vi "AccessData.vi"(0 "Vibration_Channel4_FFT":refnum<queue>, 1 "Vibration_Channel3_FFT":refnum<queue>, 2 "Vibration_Channel2_FFT":refnum<queue>, 3 "Vibration_Channel1_FFT":refnum<queue>, 4 "Vibration_Channel1":refnum<queue>, 5 "Vibration_Channel2":refnum<queue>, 6 "Vibration_Channel3":refnum<queue>, 7 "Vibration_Channel4":refnum<queue>, 8 "created path":path, 9 "Speed_Channel":refnum<queue>, 10 "IP地址":string, 12 "PRE_Scaler":u8, 14 "SAVE?":bool, 16 "Sensitivity":u16=6554, 18 "Run":refnum<queue>, 20 "Temperature_Channel1":refnum<queue>, 21 "Temperature_Channel2":refnum<queue>, 22 "Temperature_Channel3":refnum<queue>, 23 "Temperature_Channel4":refnum<queue>, 24 "Temperature_Channel5":refnum<queue>, 25 "Temperature_Channel6":refnum<queue>, 26 "Temperature_Channel7":refnum<queue>, 27 "Humidity_Channel":refnum<queue>) -> ()   [LabVIEW 2012]
uses:
  <vilib>/Analysis/NI_AALPro.lvlib
panel:
  out "系统时间":string
  out "收包":i32
  out "KB/s":dbl
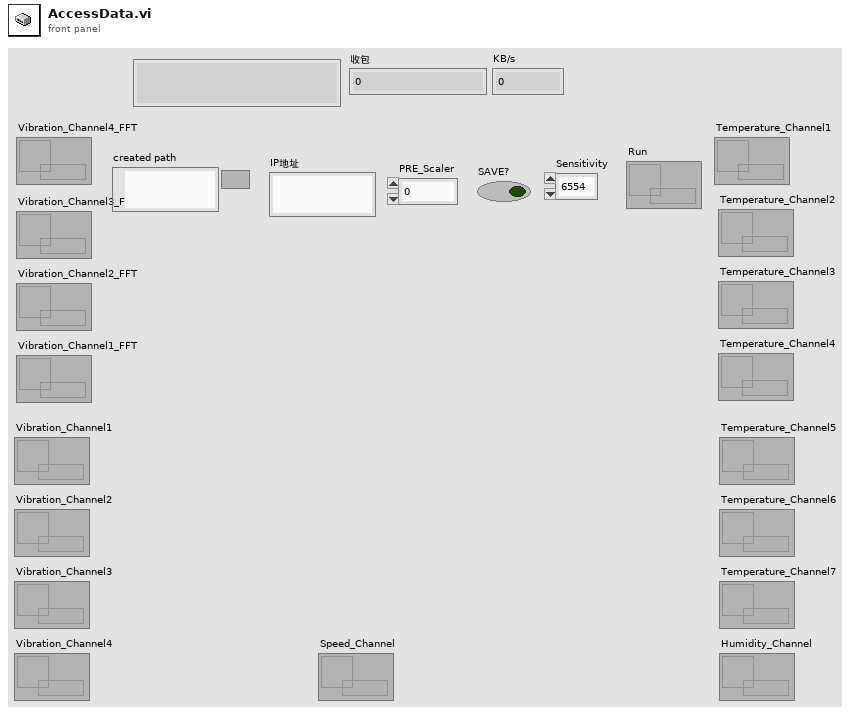
[diagram p1: front panel]
types:
  T1 = enum16{"open", "replace", "create", "open or create", "replace or create", "replace or create with confirmation"}
  T2 = enum16{"big-endian, network order", "native, host order", "little-endian"}
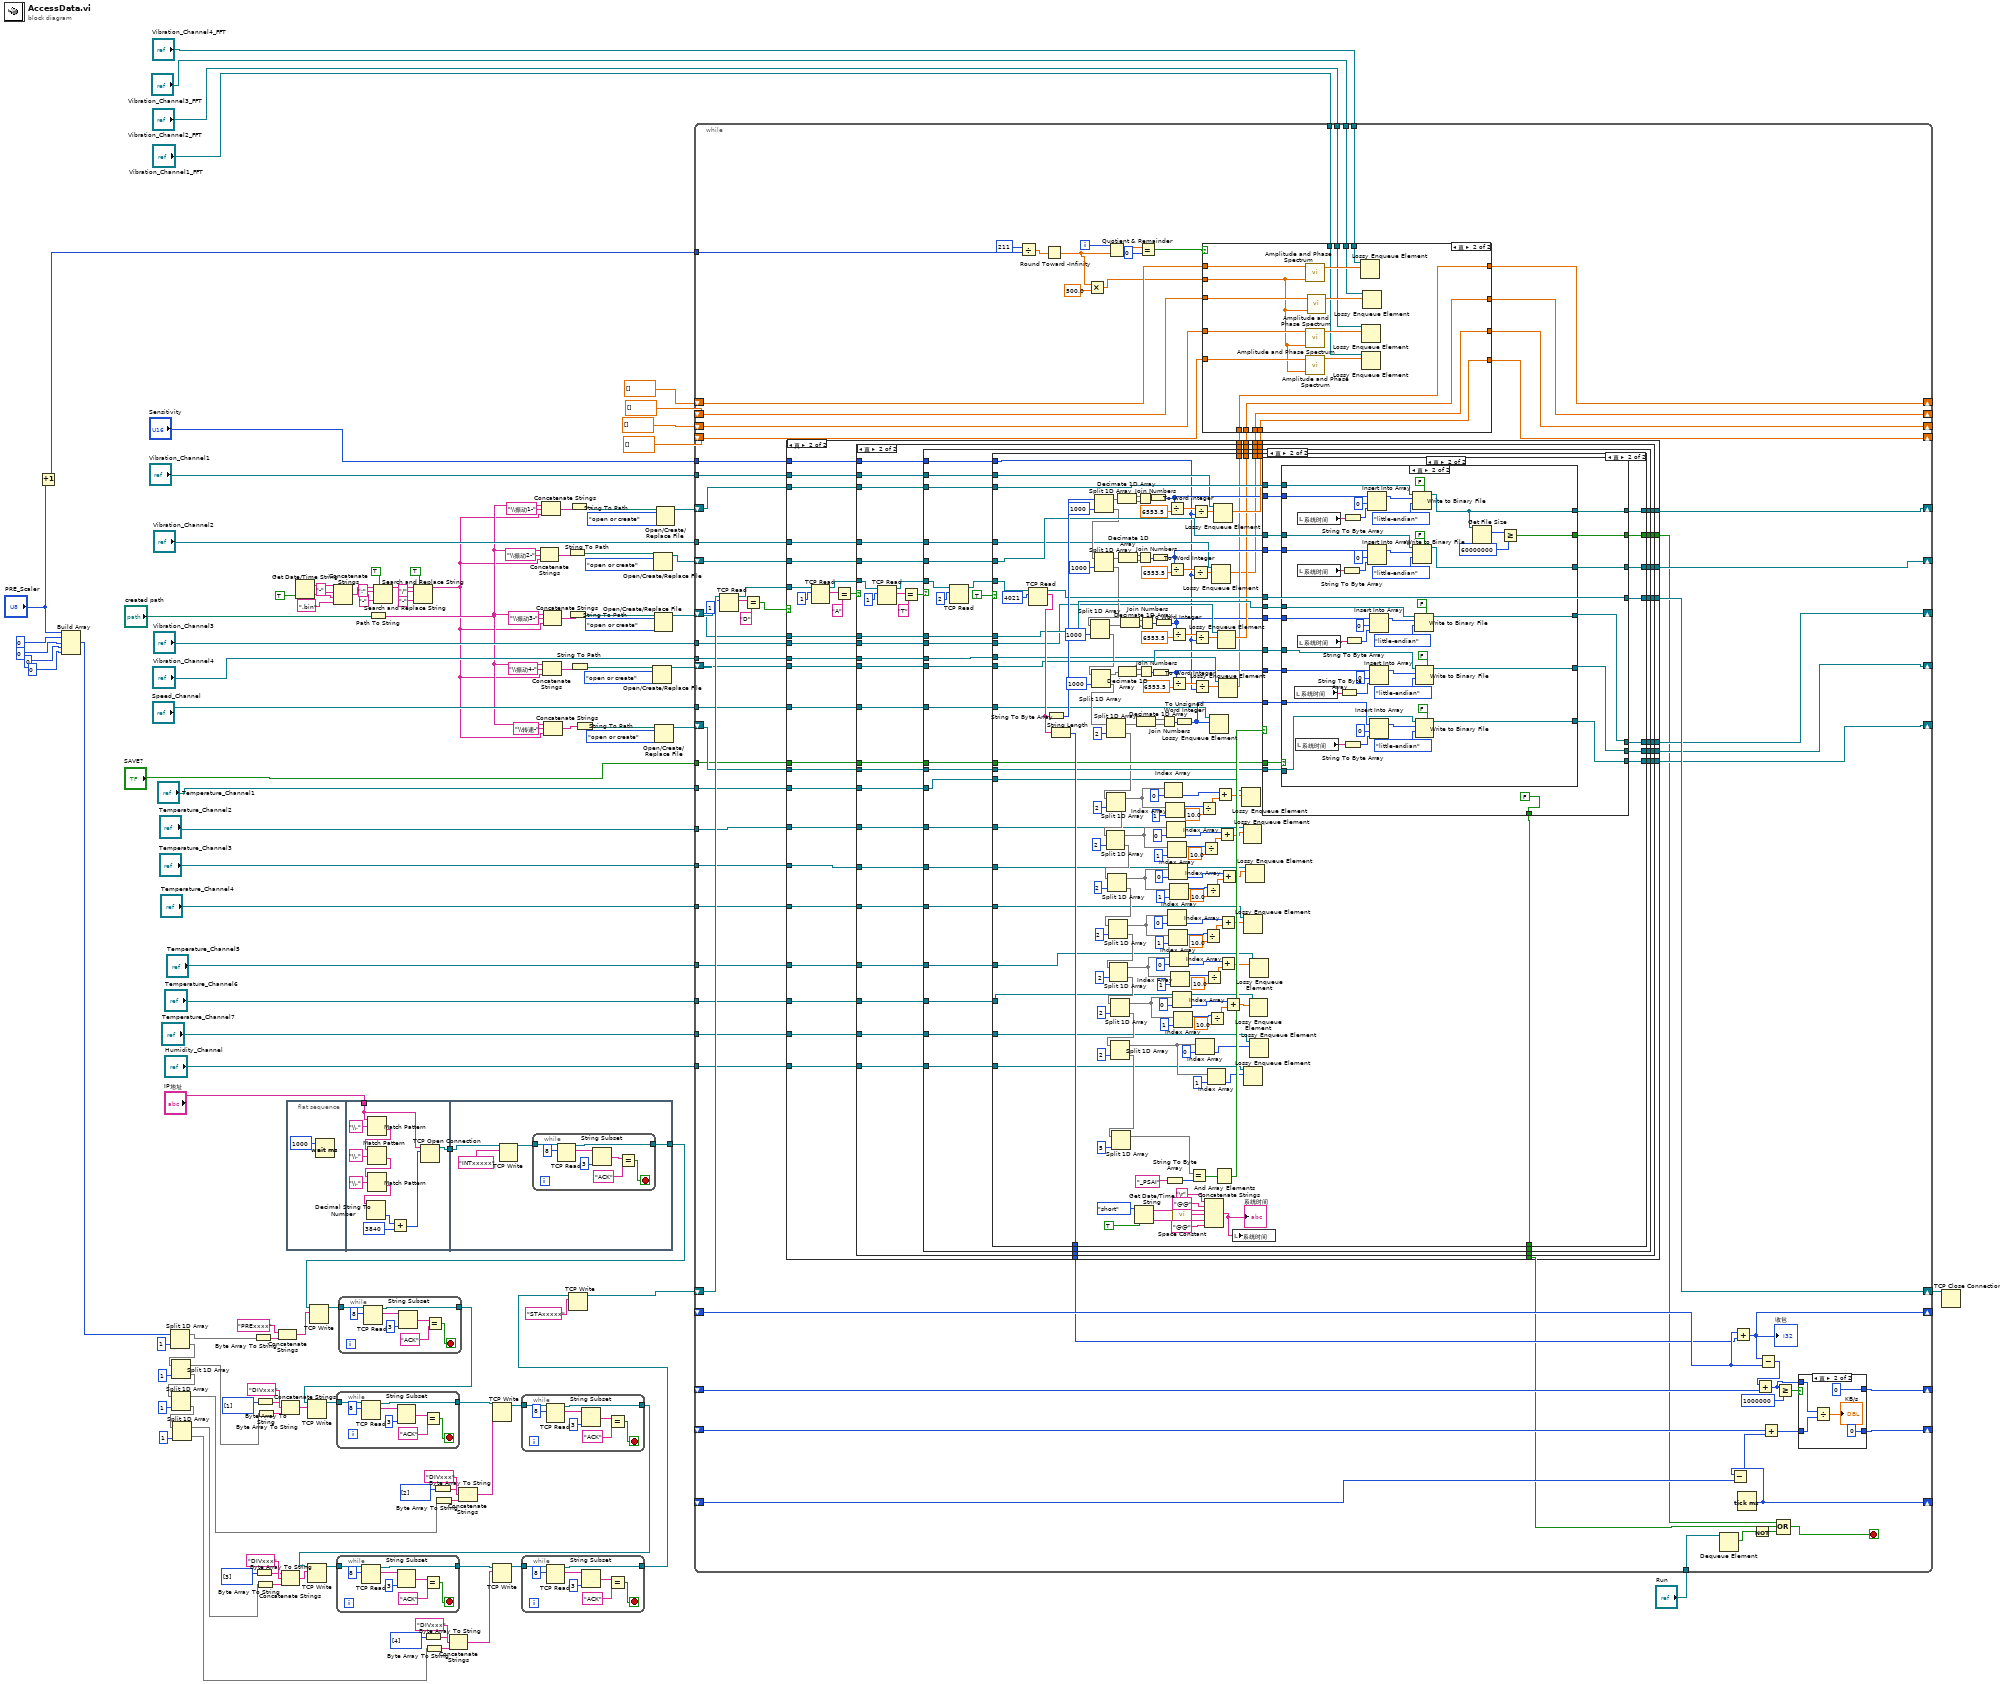
[diagram p0: block diagram]
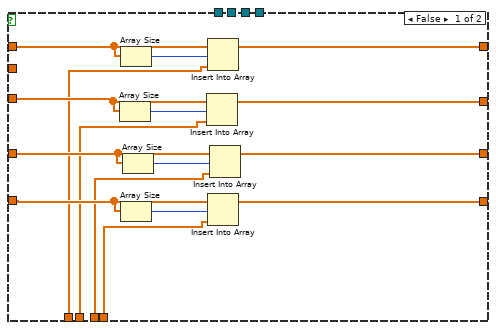
[diagram p2: hidden frame]
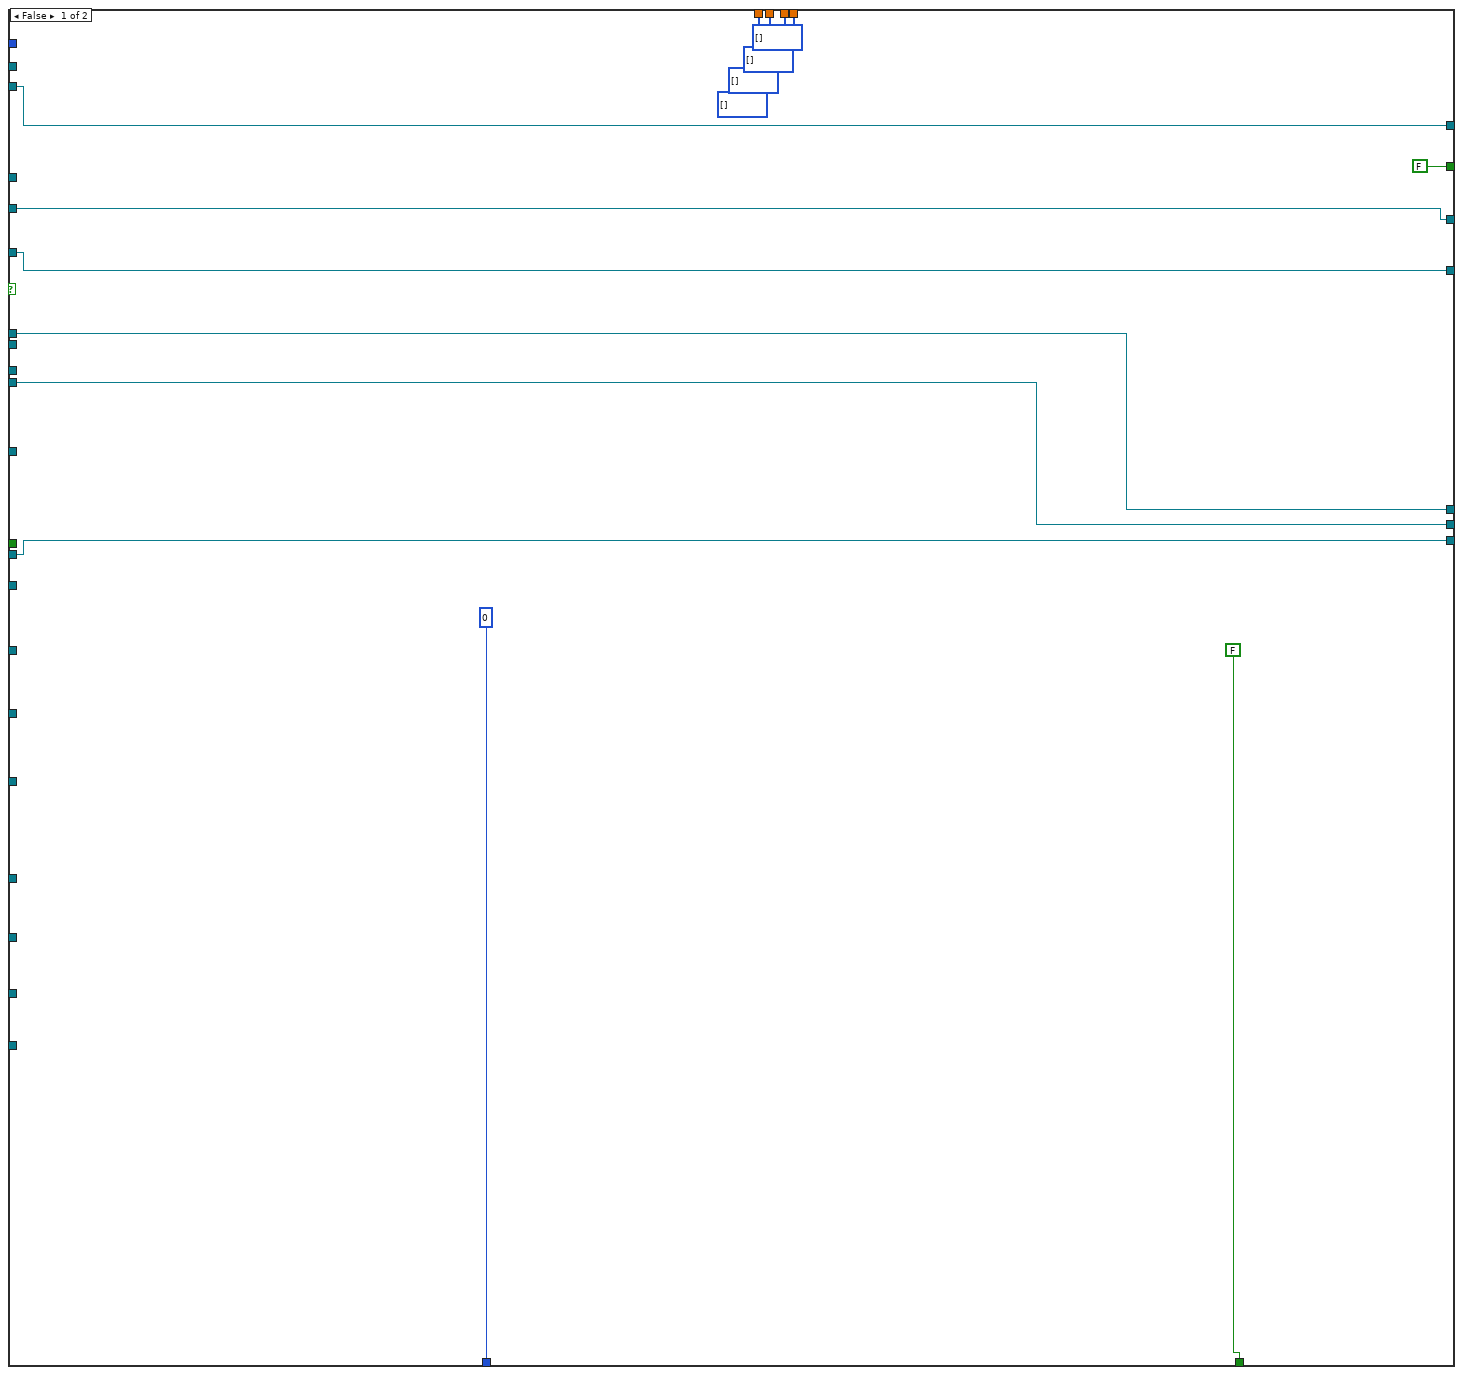
[diagram p3: hidden frame]
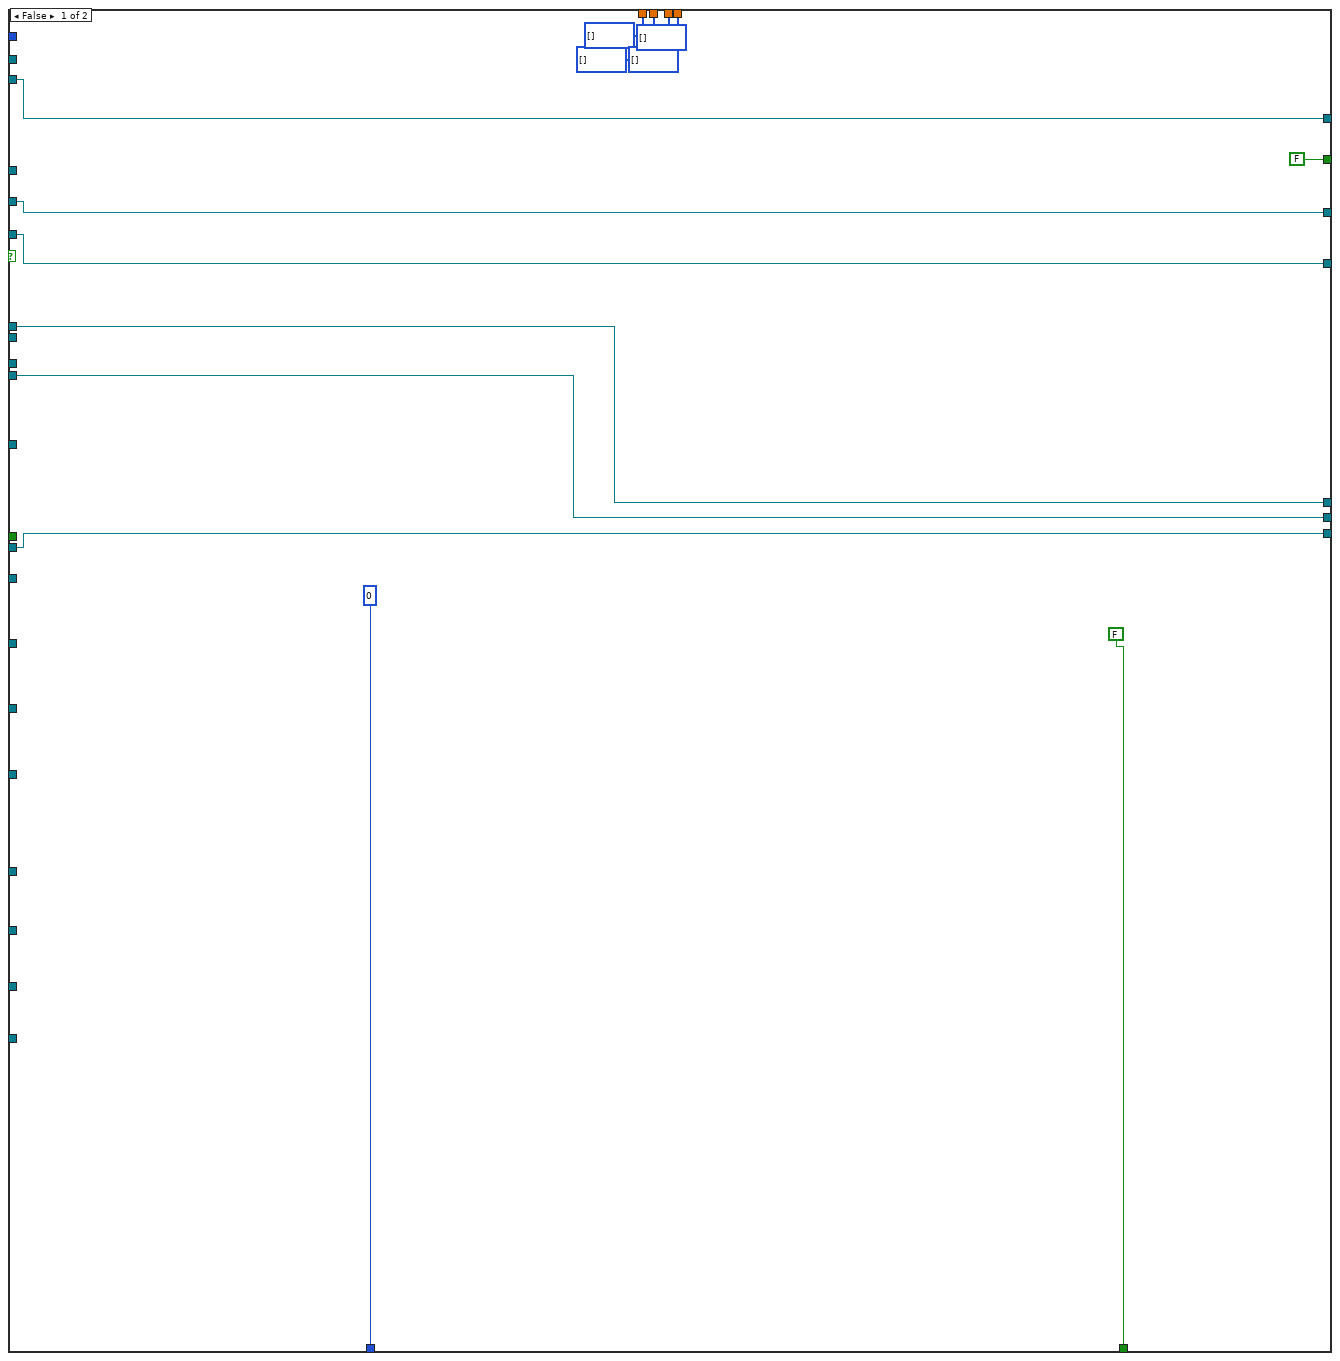
[diagram p4: hidden frame]
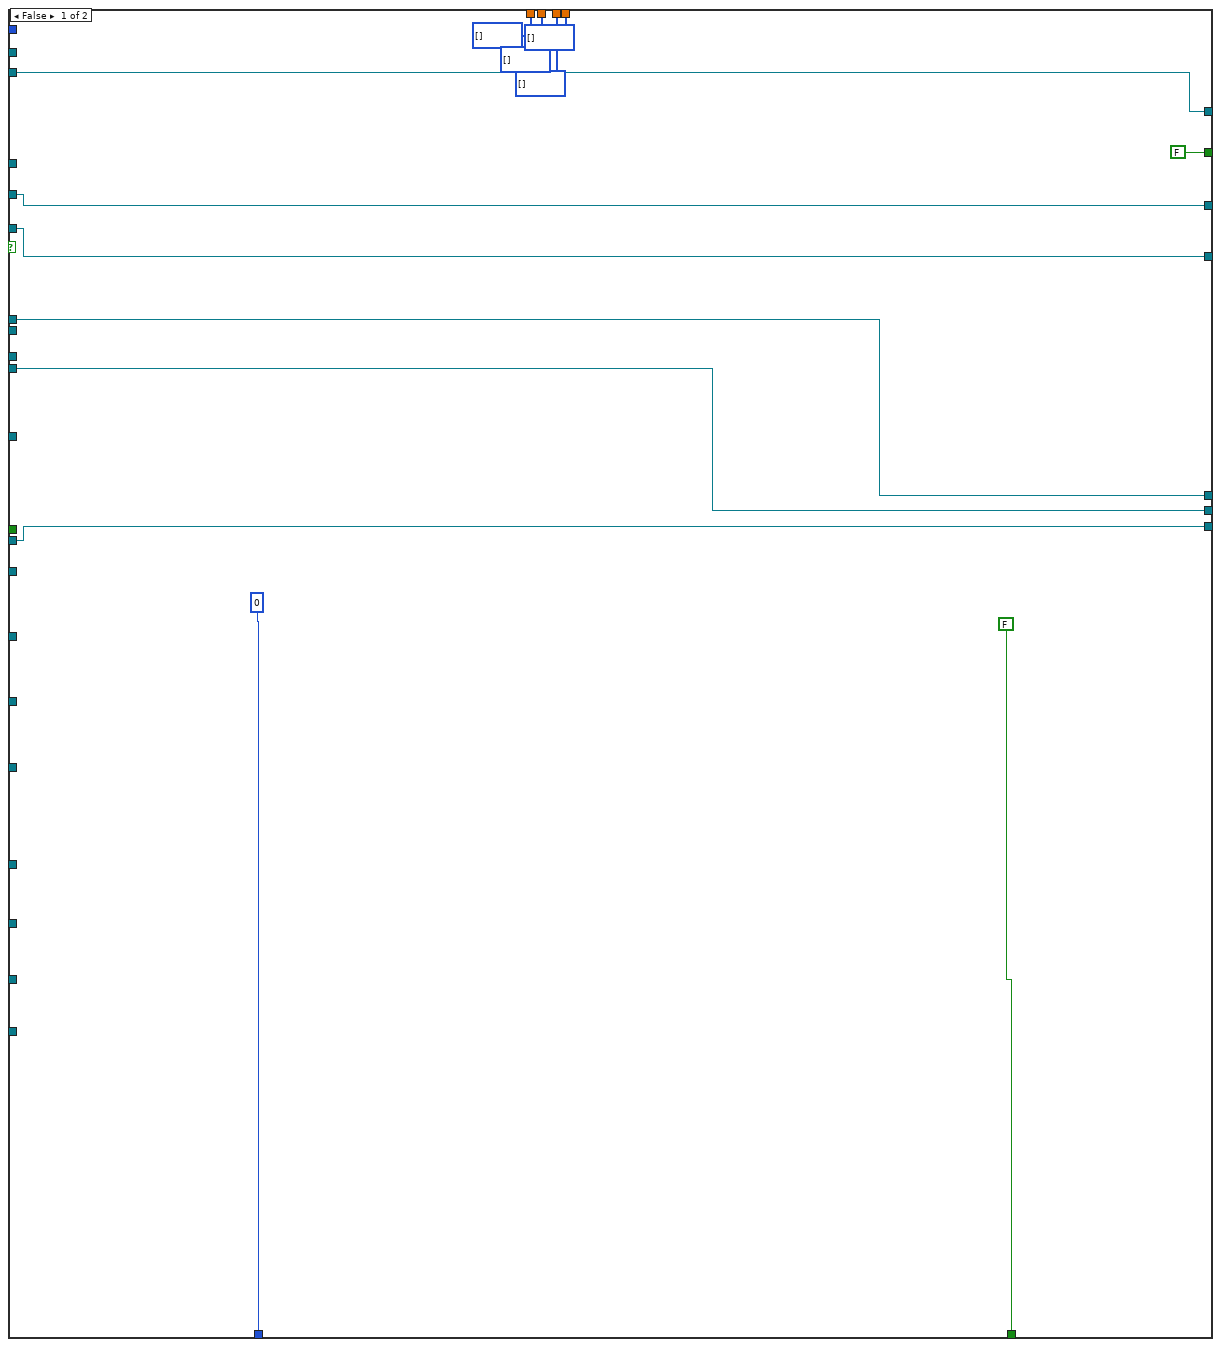
[diagram p5: hidden frame]
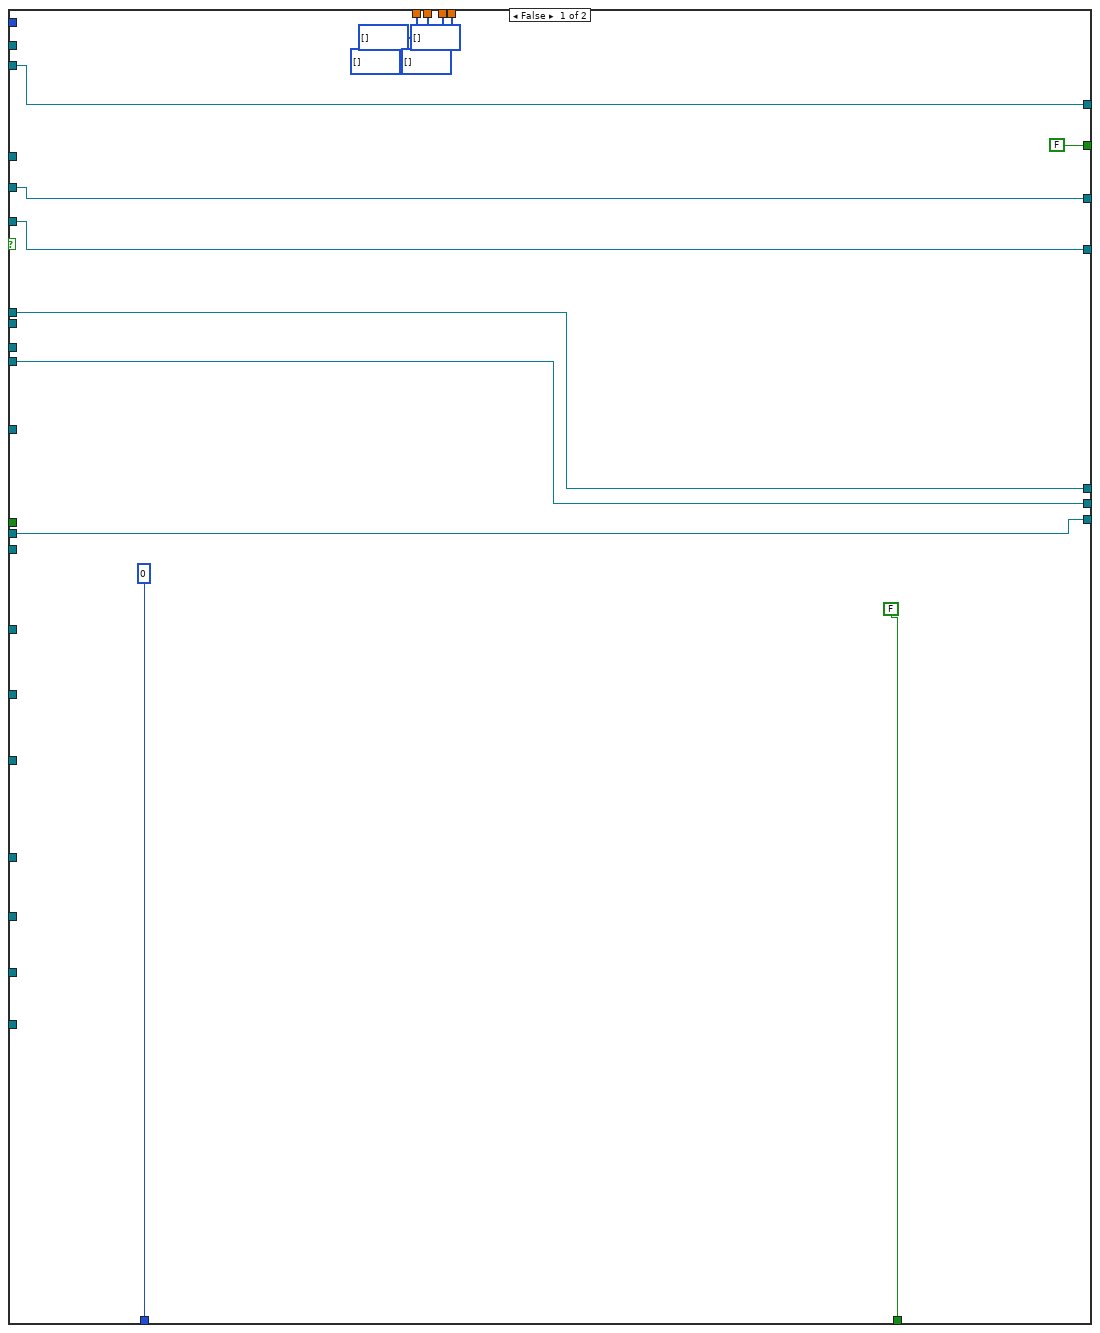
[diagram p6: hidden frame]
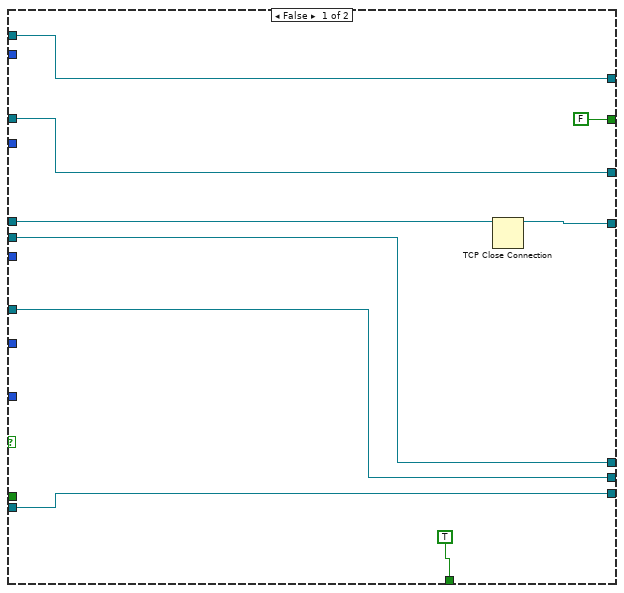
[diagram p7: hidden frame]
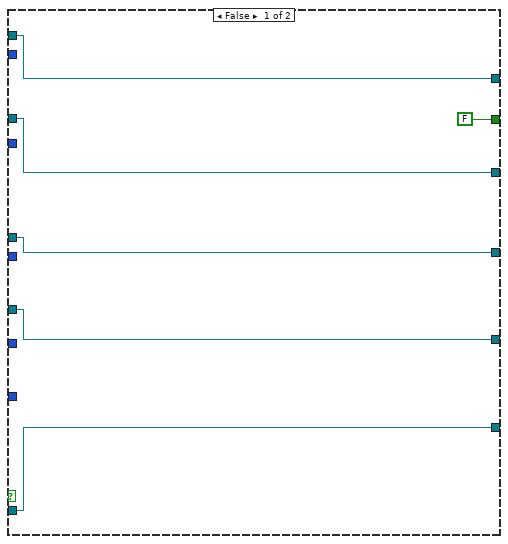
[diagram p8: hidden frame]
diagram:
  n1 = Increment(x="PRE_Scaler") -> (x+1=w101:u8)
  n2 = Build Array("PRE_Scaler", u8 0 ("元素"), u8 0 ("元素"), u8 0 ("元素"), u8 0 ("元素")) -> (w122:u8[])
  n3 = Split 1D Array(array=w122, index=1 ("索引")) -> (first subarray=w81:u8[], second subarray=w77:u8[])
  n4 = Split 1D Array(array=w77, index=1 ("索引")) -> (first subarray=w57:u8[], second subarray=w76:u8[])
  n5 = Split 1D Array(array=w76, index=1 ("索引")) -> (first subarray=w56:u8[], second subarray=w75:u8[])
  n6 = Split 1D Array(array=w75, index=1 ("索引")) -> (first subarray=w55:u8[], second subarray=w54:u8[])
  n7 = Byte Array To String(unsigned byte array=w81) -> (string=w85:string)
  n8 = Byte Array To String(unsigned byte array=u8[] [3] ("无符号字节数组")) -> (string=w63:string)
  n9 = Byte Array To String(unsigned byte array=u8[] [1] ("无符号字节数组")) -> (string=w71:string)
  n10 = Byte Array To String(unsigned byte array=w55) -> (string=w65:string)
  n11 = Byte Array To String(unsigned byte array=w57) -> (string=w74:string)
  n12 = Concatenate Strings("PRExxxx" ("数据输入"), w85) -> (w83:string)
  n13 = Concatenate Strings("DIVxxx" ("数据输入"), w71, w74) -> (w73:string)
  n14 = Concatenate Strings("DIVxxx" ("数据输入"), w63, w65) -> (w48:string)
  n15 = flat-sequence {
    tunnel: [w135] -> w123
    tunnel: "IP地址" -> [w126]
    tunnel: w123 -> [w138]
    tunnel: [w136] -> w47
    frame #0 {
      n16 = Wait (ms)(milliseconds to wait=u32 1000 ("毫秒倍数")) -> ()  [unwired: 1 out]
    }
    frame #1 {
      n17 = Match Pattern(string=w126, regular expression="\\." ("正则表达式")) -> (after substring=w130:string)  [unwired: 1 in, 3 out]
      n18 = Match Pattern(string=w130, regular expression="\\." ("正则表达式")) -> (after substring=w131:string)  [unwired: 1 in, 3 out]
      n19 = Match Pattern(string=w131, regular expression="\\." ("正则表达式")) -> (after substring=w132:string)  [unwired: 1 in, 3 out]
      n20 = Decimal String To Number(string=w132) -> (number=w133:i32)  [unwired: 2 in, 1 out]
      n21 = Add(x=w133, y=3840) -> (x+y=w125:i32)
      n22 = TCP Open Connection(address=w126, remote port or service name=w125) -> (connection ID=w135:refnum<k5>)  [unwired: 3 in, 1 out]
    }
    frame #2 {
      n23 = TCP Write(connection ID=w138, data in="INTxxxxx" ("数据输入")) -> (connection ID out=w137:refnum<k5>)  [unwired: 2 in, 2 out]
      n24 = while {
        tunnel: w137 -> [w147]
        tunnel: [w141] -> w136
        stop <- w142 stop-if-true
        n25 = TCP Read(connection ID=w147, bytes to read=8 ("读取的字节")) -> (connection ID out=w141:refnum<k5>, data out=w145:string)  [unwired: 3 in, 1 out]
        n26 = String Subset(string=w145, length (rest)=3 ("偏移量(0)")) -> (substring=w144:string)  [unwired: 1 in]
        n27 = Equal?(x=w144, y="ACK") -> (x = y?=w142:bool)
      }
    }
  }
  n28 = Get Date/Time String(want seconds? (F)=TRUE ("需要秒？(F)")) -> (date string=w19:string, time string=w16:string)  [unwired: 2 in]
  n29 = TCP Write(connection ID=w47, data in=w83) -> (connection ID out=w94:refnum<k5>)  [unwired: 2 in, 2 out]
  n30 = Concatenate Strings(w19, "-" ("字符串"), w16, ".bin" ("字符串")) -> (w15:string)
  n31 = while {
    tunnel: w94 -> [w155]
    tunnel: [w149] -> w89
    stop <- w150 stop-if-true
    n32 = TCP Read(connection ID=w155, bytes to read=8 ("读取的字节")) -> (connection ID out=w149:refnum<k5>, data out=w153:string)  [unwired: 3 in, 1 out]
    n33 = String Subset(string=w153, length (rest)=3 ("偏移量(0)")) -> (substring=w152:string)  [unwired: 1 in]
    n34 = Equal?(x=w152, y="ACK") -> (x = y?=w150:bool)
  }
  n35 = TCP Write(connection ID=w89, data in=w73) -> (connection ID out=w93:refnum<k5>)  [unwired: 2 in, 2 out]
  n36 = while {
    tunnel: w93 -> [w163]
    tunnel: [w157] -> w88
    stop <- w158 stop-if-true
    n37 = TCP Read(connection ID=w163, bytes to read=8 ("读取的字节")) -> (connection ID out=w157:refnum<k5>, data out=w161:string)  [unwired: 3 in, 1 out]
    n38 = String Subset(string=w161, length (rest)=3 ("偏移量(0)")) -> (substring=w160:string)  [unwired: 1 in]
    n39 = Equal?(x=w160, y="ACK") -> (x = y?=w158:bool)
  }
  n40 = Path To String(path="created path") -> (string=w31:string)
  n41 = Search and Replace String(replace all?=TRUE ("替换全部？(F)"), input string=w15, search string=":" ("搜索字符串"), replace string="-" ("替换字符串(\"\")")) -> (result string=w8:string)  [unwired: 4 in, 3 out]
  n42 = Search and Replace String(replace all?=TRUE ("替换全部？(F)"), input string=w8, search string="/" ("搜索字符串"), replace string="-" ("替换字符串(\"\")")) -> (result string=w7:string)  [unwired: 4 in, 3 out]
  n43 = Byte Array To String(unsigned byte array=u8[] [4] ("无符号字节数组")) -> (string=w59:string)
  n44 = Byte Array To String(unsigned byte array=w54) -> (string=w61:string)
  n45 = Byte Array To String(unsigned byte array=u8[] [2] ("无符号字节数组")) -> (string=w67:string)
  n46 = Byte Array To String(unsigned byte array=w56) -> (string=w69:string)
  n47 = Concatenate Strings("DIVxxx" ("数据输入"), w59, w61) -> (w52:string)
  n48 = Concatenate Strings("DIVxxx" ("数据输入"), w67, w69) -> (w53:string)
  n49 = TCP Write(connection ID=w88, data in=w53) -> (connection ID out=w92:refnum<k5>)  [unwired: 2 in, 2 out]
  n50 = while {
    tunnel: w92 -> [w171]
    tunnel: [w165] -> w87
    stop <- w166 stop-if-true
    n51 = TCP Read(connection ID=w171, bytes to read=8 ("读取的字节")) -> (connection ID out=w165:refnum<k5>, data out=w169:string)  [unwired: 3 in, 1 out]
    n52 = String Subset(string=w169, length (rest)=3 ("偏移量(0)")) -> (substring=w168:string)  [unwired: 1 in]
    n53 = Equal?(x=w168, y="ACK") -> (x = y?=w166:bool)
  }
  n54 = TCP Write(connection ID=w87, data in=w48) -> (connection ID out=w91:refnum<k5>)  [unwired: 2 in, 2 out]
  n55 = while {
    tunnel: w91 -> [w179]
    tunnel: [w173] -> w86
    stop <- w174 stop-if-true
    n56 = TCP Read(connection ID=w179, bytes to read=8 ("读取的字节")) -> (connection ID out=w173:refnum<k5>, data out=w177:string)  [unwired: 3 in, 1 out]
    n57 = String Subset(string=w177, length (rest)=3 ("偏移量(0)")) -> (substring=w176:string)  [unwired: 1 in]
    n58 = Equal?(x=w176, y="ACK") -> (x = y?=w174:bool)
  }
  n59 = TCP Write(connection ID=w86, data in=w52) -> (connection ID out=w90:refnum<k5>)  [unwired: 2 in, 2 out]
  n60 = while {
    tunnel: w90 -> [w187]
    tunnel: [w181] -> w51
    stop <- w182 stop-if-true
    n61 = TCP Read(connection ID=w187, bytes to read=8 ("读取的字节")) -> (connection ID out=w181:refnum<k5>, data out=w185:string)  [unwired: 3 in, 1 out]
    n62 = String Subset(string=w185, length (rest)=3 ("偏移量(0)")) -> (substring=w184:string)  [unwired: 1 in]
    n63 = Equal?(x=w184, y="ACK") -> (x = y?=w182:bool)
  }
  n64 = Concatenate Strings(w31, "\\振动2-" ("字符串"), w7) -> (w38:string)
  n65 = Concatenate Strings(w31, "\\振动1-" ("字符串"), w7) -> (w37:string)
  n66 = Concatenate Strings(w31, "\\振动4-" ("字符串"), w7) -> (w40:string)
  n67 = Concatenate Strings(w31, "\\振动3-" ("字符串"), w7) -> (w39:string)
  n68 = Concatenate Strings(w31, "\\转速-" ("字符串"), w7) -> (w41:string)
  n69 = String To Path(string=w38) -> (path=w35:path)
  n70 = String To Path(string=w39) -> (path=w34:path)
  n71 = TCP Write(connection ID=w51, data in="STAxxxxx" ("数据输入")) -> (connection ID out=w49:refnum<k5>)  [unwired: 2 in, 2 out]
  n72 = String To Path(string=w37) -> (path=w36:path)
  n73 = String To Path(string=w40) -> (path=w33:path)
  n74 = String To Path(string=w41) -> (path=w32:path)
  n75 = Open/Create/Replace File(file path (use dialog)=w33, operation (0:open)=T1."open or create" ("操作(0:open)")) -> (refnum out=w22:refnum<file>)  [unwired: 4 in, 2 out]
  n76 = Open/Create/Replace File(file path (use dialog)=w35, operation (0:open)=T1."open or create" ("操作(0:open)")) -> (refnum out=w24:refnum<file>)  [unwired: 4 in, 2 out]
  n77 = Open/Create/Replace File(file path (use dialog)=w34, operation (0:open)=T1."open or create" ("操作(0:open)")) -> (refnum out=w23:refnum<file>)  [unwired: 4 in, 2 out]
  n78 = Open/Create/Replace File(file path (use dialog)=w32, operation (0:open)=T1."open or create" ("操作(0:open)")) -> (refnum out=w21:refnum<file>)  [unwired: 4 in, 2 out]
  n79 = Open/Create/Replace File(file path (use dialog)=w36, operation (0:open)=T1."open or create" ("操作(0:open)")) -> (refnum out=w25:refnum<file>)  [unwired: 4 in, 2 out]
  n80 = while {
    shift-right: [w266] -> _
    shift-left: _ -> [w265]
    shift-right: [w248] -> w2
    shift-left: w49 -> [w252]
    shift-right: [w260] -> _
    shift-left: _ -> [w263]
    shift-right: [w257] -> _
    shift-left: _ -> [w258]
    shift-right: [w255] -> _
    shift-left: _ -> [w253]
    shift-right: [w244] -> _
    shift-left: w25 -> [w239]
    shift-right: [w243] -> _
    shift-left: w24 -> [w238]
    shift-right: [w242] -> _
    shift-left: w23 -> [w237]
    shift-right: [w241] -> _
    shift-left: w22 -> [w236]
    shift-right: [w240] -> _
    shift-left: w21 -> [w235]
    tunnel: "SAVE?" -> [w234]
    shift-right: [w219] -> _
    shift-left: dbl[] [] -> [w223]
    shift-right: [w220] -> _
    shift-left: dbl[] [] -> [w224]
    shift-right: [w221] -> _
    shift-left: dbl[] [] -> [w225]
    shift-right: [w222] -> _
    shift-left: dbl[] [] -> [w218]
    tunnel: w101 -> [w214]
    tunnel: "Vibration_Channel1" -> [w211]
    tunnel: "Vibration_Channel2" -> [w210]
    tunnel: "Vibration_Channel3" -> [w209]
    tunnel: "Vibration_Channel4" -> [w208]
    tunnel: "Speed_Channel" -> [w207]
    tunnel: "Vibration_Channel4_FFT" -> [w206]
    tunnel: "Vibration_Channel3_FFT" -> [w205]
    tunnel: "Vibration_Channel2_FFT" -> [w204]
    tunnel: "Vibration_Channel1_FFT" -> [w203]
    tunnel: "Temperature_Channel1" -> [w202]
    tunnel: "Temperature_Channel2" -> [w201]
    tunnel: "Temperature_Channel3" -> [w200]
    tunnel: "Temperature_Channel4" -> [w199]
    tunnel: "Temperature_Channel5" -> [w198]
    tunnel: "Temperature_Channel6" -> [w197]
    tunnel: "Temperature_Channel7" -> [w196]
    tunnel: "Humidity_Channel" -> [w195]
    tunnel: "Sensitivity" -> [w194]
    tunnel: "Run" -> [w188]
    i -> [w233]
    stop <- w193 stop-if-true
    n81 = TCP Read(connection ID=w252, bytes to read=1 ("读取的字节")) -> (connection ID out=w245:refnum<k5>, data out=w250:string)  [unwired: 3 in, 1 out]
    n82 = Equal?(x=w250, y="D") -> (x = y?=w246:bool)
    n83 = case shown="真" w246 {
      tunnel: w245 -> [w312 w347]
      tunnel: [w312 w346] -> w248
      tunnel: [0 w345] -> w247
      tunnel: [FALSE w343] -> w191
      tunnel: [w309 w342] -> w244
      tunnel: [w308 w335] -> w243
      tunnel: [w307 w334] -> w242
      tunnel: [w306 w333] -> w241
      tunnel: [w305 w341] -> w240
      tunnel: w239 -> [w309 w340]
      tunnel: w238 -> [w308 w339]
      tunnel: w237 -> [w307 w338]
      tunnel: w236 -> [w306 w337]
      tunnel: w235 -> [w305 w336]
      tunnel: w234 -> [_ w332]
      tunnel: [FALSE w331] -> w192
      tunnel: [i16[] [] w330] -> w229
      tunnel: [i16[] [] w329] -> w228
      tunnel: [i16[] [] w328] -> w227
      tunnel: [i16[] [] w327] -> w226
      tunnel: w211 -> [_ w326]
      tunnel: w210 -> [_ w325]
      tunnel: w209 -> [_ w324]
      tunnel: w208 -> [_ w323]
      tunnel: w207 -> [_ w322]
      tunnel: w202 -> [_ w321]
      tunnel: w201 -> [_ w320]
      tunnel: w200 -> [_ w319]
      tunnel: w199 -> [_ w318]
      tunnel: w198 -> [_ w317]
      tunnel: w197 -> [_ w316]
      tunnel: w196 -> [_ w315]
      tunnel: w195 -> [_ w314]
      tunnel: w194 -> [_ w313]
      frame False {
      }
      frame True {
        n84 = TCP Read(connection ID=w347, bytes to read=1 ("读取的字节")) -> (connection ID out=w344:refnum<k5>, data out=w350:string)  [unwired: 3 in, 1 out]
        n85 = Equal?(x=w350, y="A") -> (x = y?=w348:bool)
        n86 = case shown="真" w348 {
          tunnel: w344 -> [w364 w399]
          tunnel: [w364 w398] -> w346
          tunnel: [0 w397] -> w345
          tunnel: [FALSE w395] -> w343
          tunnel: [w361 w394] -> w342
          tunnel: [w357 w390] -> w341
          tunnel: w340 -> [w361 w389]
          tunnel: w339 -> [w360 w388]
          tunnel: w338 -> [w359 w387]
          tunnel: w337 -> [w358 w386]
          tunnel: w336 -> [w357 w385]
          tunnel: [w360 w393] -> w335
          tunnel: [w359 w392] -> w334
          tunnel: [w358 w391] -> w333
          tunnel: w332 -> [_ w384]
          tunnel: [FALSE w383] -> w331
          tunnel: [i16[] [] w382] -> w330
          tunnel: [i16[] [] w381] -> w329
          tunnel: [i16[] [] w380] -> w328
          tunnel: [i16[] [] w379] -> w327
          tunnel: w326 -> [_ w378]
          tunnel: w325 -> [_ w377]
          tunnel: w324 -> [_ w376]
          tunnel: w323 -> [_ w375]
          tunnel: w322 -> [_ w374]
          tunnel: w321 -> [_ w373]
          tunnel: w320 -> [_ w372]
          tunnel: w319 -> [_ w371]
          tunnel: w318 -> [_ w370]
          tunnel: w317 -> [_ w369]
          tunnel: w316 -> [_ w368]
          tunnel: w315 -> [_ w367]
          tunnel: w314 -> [_ w366]
          tunnel: w313 -> [_ w365]
          frame False {
          }
          frame True {
            n87 = TCP Read(connection ID=w399, bytes to read=1 ("读取的字节")) -> (connection ID out=w396:refnum<k5>, data out=w402:string)  [unwired: 3 in, 1 out]
            n88 = Equal?(x=w402, y="T") -> (x = y?=w400:bool)
            n89 = case shown="真" w400 {
              tunnel: w396 -> [w416 w452]
              tunnel: [w416 w449] -> w398
              tunnel: [0 w451] -> w397
              tunnel: [FALSE w448] -> w395
              tunnel: [w409 w440] -> w394
              tunnel: [w410 w439] -> w393
              tunnel: [w411 w438] -> w392
              tunnel: [w412 w447] -> w391
              tunnel: [w413 w446] -> w390
              tunnel: w389 -> [w409 w445]
              tunnel: w388 -> [w410 w444]
              tunnel: w387 -> [w411 w443]
              tunnel: w386 -> [w412 w442]
              tunnel: w385 -> [w413 w441]
              tunnel: w384 -> [_ w437]
              tunnel: [FALSE w436] -> w383
              tunnel: [i16[] [] w435] -> w382
              tunnel: [i16[] [] w434] -> w381
              tunnel: [i16[] [] w433] -> w380
              tunnel: [i16[] [] w432] -> w379
              tunnel: w378 -> [_ w430]
              tunnel: w377 -> [_ w429]
              tunnel: w376 -> [_ w428]
              tunnel: w375 -> [_ w427]
              tunnel: w374 -> [_ w426]
              tunnel: w373 -> [_ w425]
              tunnel: w372 -> [_ w424]
              tunnel: w371 -> [_ w423]
              tunnel: w370 -> [_ w422]
              tunnel: w369 -> [_ w421]
              tunnel: w368 -> [_ w420]
              tunnel: w367 -> [_ w419]
              tunnel: w366 -> [_ w418]
              tunnel: w365 -> [_ w417]
              frame False {
              }
              frame True {
                n90 = TCP Read(connection ID=w452, bytes to read=2 ("读取的字节")) -> (connection ID out=w450:refnum<k5>)  [unwired: 3 in, 2 out]
                n91 = case shown="真" TRUE {
                  tunnel: w450 -> [w466 w628]
                  tunnel: [0 w619] -> w451
                  tunnel: [w466 w612] -> w449
                  tunnel: [FALSE w613] -> w448
                  tunnel: [w460 w595] -> w447
                  tunnel: [w459 w594] -> w446
                  tunnel: w445 -> [w463 w601]
                  tunnel: w444 -> [w462 w599]
                  tunnel: w443 -> [w461 w597]
                  tunnel: w442 -> [w460 w529]
                  tunnel: w441 -> [w459 w593]
                  tunnel: [w463 w600] -> w440
                  tunnel: [w462 w598] -> w439
                  tunnel: [w461 w596] -> w438
                  tunnel: w437 -> [_ w591]
                  tunnel: [FALSE w589] -> w436
                  tunnel: [i16[] [] w483] -> w435
                  tunnel: [i16[] [] w473] -> w434
                  tunnel: [i16[] [] w477] -> w433
                  tunnel: [i16[] [] w475] -> w432
                  tunnel: w430 -> [_ w504]
                  tunnel: w429 -> [_ w472]
                  tunnel: w428 -> [_ w503]
                  tunnel: w427 -> [_ w502]
                  tunnel: w426 -> [_ w501]
                  tunnel: w425 -> [_ w494]
                  tunnel: w424 -> [_ w493]
                  tunnel: w423 -> [_ w492]
                  tunnel: w422 -> [_ w491]
                  tunnel: w421 -> [_ w490]
                  tunnel: w420 -> [_ w489]
                  tunnel: w419 -> [_ w486]
                  tunnel: w418 -> [_ w485]
                  tunnel: w417 -> [_ w467]
                  frame False {
                  }
                  frame True {
                    n92 = TCP Read(connection ID=w628, bytes to read=4021 ("最大值(548)")) -> (connection ID out=w602:refnum<k5>, data out=w611:string)  [unwired: 3 in, 1 out]
                    n93 = String To Byte Array(string=w611) -> (unsigned byte array=w610:u8[])
                    n94 = String Length(string=w611) -> (length=w619:i32)
                    n95 = Split 1D Array(array=w610, index=1000 ("索引")) -> (first subarray=w527:u8[], second subarray=w524:u8[])
                    n96 = Split 1D Array(array=w524, index=1000 ("索引")) -> (first subarray=w523:u8[], second subarray=w520:u8[])
                    n97 = Split 1D Array(array=w520, index=1000 ("索引")) -> (first subarray=w519:u8[], second subarray=w518:u8[])
                    n98 = Split 1D Array(array=w518, index=1000 ("索引")) -> (first subarray=w515:u8[], second subarray=w528:u8[])
                    n99 = Split 1D Array(array=w528, index=2 ("索引")) -> (first subarray=w512:u8[], second subarray=w588:u8[])
                    n100 = Split 1D Array(array=w588, index=2 ("索引")) -> (first subarray=w571:u8[], second subarray=w587:u8[])
                    n101 = Split 1D Array(array=w587, index=2 ("索引")) -> (first subarray=w535:u8[], second subarray=w586:u8[])
                    n102 = Split 1D Array(array=w586, index=2 ("索引")) -> (first subarray=w534:u8[], second subarray=w573:u8[])
                    n103 = Split 1D Array(array=w573, index=2 ("索引")) -> (first subarray=w533:u8[], second subarray=w582:u8[])
                    n104 = Split 1D Array(array=w582, index=2 ("索引")) -> (first subarray=w532:u8[], second subarray=w581:u8[])
                    n105 = Split 1D Array(array=w581, index=2 ("索引")) -> (first subarray=w531:u8[], second subarray=w572:u8[])
                    n106 = Split 1D Array(array=w572, index=2 ("索引")) -> (first subarray=w530:u8[], second subarray=w507:u8[])
                    n107 = Split 1D Array(array=w507, index=5 ("索引")) -> (first subarray=w506:u8[])  [unwired: 1 out]
                    n108 = Decimate 1D Array(w527) -> (w526:u8[], w525:u8[])
                    n109 = Decimate 1D Array(w515) -> (w514:u8[], w513:u8[])
                    n110 = Decimate 1D Array(w523) -> (w522:u8[], w521:u8[])
                    n111 = Decimate 1D Array(w519) -> (w517:u8[], w516:u8[])
                    n112 = Get Date/Time String(date format (0)=enum16{"short", "long", "abbreviated"}."short" ("日期格式(0)"), want seconds? (F)=TRUE ("需要秒？(F)")) -> (date string=w607:string, time string=w590:string)  [unwired: 1 in]
                    n113 = Join Numbers(hi=w526, lo=w525) -> ((hi.lo)=w626:u16[])
                    n114 = Join Numbers(hi=w522, lo=w521) -> ((hi.lo)=w621:u16[])
                    n115 = Decimate 1D Array(w512) -> (w511:u8[], w510:u8[])
                    n116 = Join Numbers(hi=w514, lo=w513) -> ((hi.lo)=w623:u16[])
                    n117 = Join Numbers(hi=w517, lo=w516) -> ((hi.lo)=w622:u16[])
                    n118 = To Word Integer(number=w626) -> (16bit integer=w482:i16[])
                    n119 = To Word Integer(number=w621) -> (16bit integer=w478:i16[])
                    n120 = To Word Integer(number=w623) -> (16bit integer=w474:i16[])
                    n121 = To Word Integer(number=w622) -> (16bit integer=w476:i16[])
                    n122 = Join Numbers(hi=w511, lo=w510) -> ((hi.lo)=w509:u16[])
                    n123 = Index Array(array=w571, index=0 ("索引")) -> (element=w566:u8)
                    n124 = Index Array(array=w571, index=1 ("索引")) -> (element=w568:u8)
                    n125 = String To Byte Array(string="_PSAI") -> (unsigned byte array=w616:u8[])
                    n126 = Index Array(array=w535, index=0 ("索引")) -> (element=w560:u8)
                    n127 = Divide(x=w482, y=6553.5) -> (x/y=w468:dbl[])
                    n128 = Divide(x=w478, y=6553.5) -> (x/y=w469:dbl[])
                    n129 = Index Array(array=w535, index=1 ("索引")) -> (element=w562:u8)
                    n130 = Index Array(array=w533, index=0 ("索引")) -> (element=w548:u8)
                    n131 = Index Array(array=w534, index=0 ("索引")) -> (element=w554:u8)
                    n132 = Index Array(array=w533, index=1 ("索引")) -> (element=w550:u8)
                    n133 = Divide(x=w476, y=6553.5) -> (x/y=w470:dbl[])
                    n134 = Divide(x=w474, y=6553.5) -> (x/y=w471:dbl[])
                    n135 = Index Array(array=w534, index=1 ("索引")) -> (element=w556:u8)
                    n136 = Index Array(array=w532, index=0 ("索引")) -> (element=w542:u8)
                    n137 = Index Array(array=w532, index=1 ("索引")) -> (element=w544:u8)
                    n138 = Index Array(array=w531, index=0 ("索引")) -> (element=w536:u8)
                    n139 = call <vilib>:"Space Constant.vi"() -> ("String"=w603:string)
                    n140 = Index Array(array=w531, index=1 ("索引")) -> (element=w538:u8)
                    n141 = To Unsigned Word Integer(number=w509) -> (unsigned 16bit integer=w505:u16[])
                    n142 = Equal?(x=w506, y=w616) -> (x = y?=w615:bool[])
                    n143 = Divide(x=w469, y=w467) -> (x/y=w473:dbl[])
                    n144 = Divide(x=w468, y=w467) -> (x/y=w483:dbl[])
                    n145 = Divide(x=w470, y=w467) -> (x/y=w477:dbl[])
                    n146 = Divide(x=w471, y=w467) -> (x/y=w475:dbl[])
                    n147 = Index Array(array=w530, index=0 ("索引")) -> (element=w488:u8)
                    n148 = Divide(x=w568, y=10.0) -> (x/y=w567:dbl)
                    n149 = Divide(x=w562, y=10.0) -> (x/y=w561:dbl)
                    n150 = Divide(x=w550, y=10.0) -> (x/y=w549:dbl)
                    n151 = Divide(x=w556, y=10.0) -> (x/y=w555:dbl)
                    n152 = Concatenate Strings("\r", "@@" ("字符串"), w607, w603, w590, "@@" ("字符串")) -> (w606:string)
                    "系统时间" <- w606
                    n153 = Divide(x=w544, y=10.0) -> (x/y=w543:dbl)
                    n154 = Index Array(array=w530, index=1 ("索引")) -> (element=w487:u8)
                    n155 = Divide(x=w538, y=10.0) -> (x/y=w537:dbl)
                    n156 = Lossy Enqueue Element(queue=w501, element=w505) -> ()  [unwired: 1 in, 4 out]
                    n157 = Lossy Enqueue Element(queue=w472, element=w473) -> ()  [unwired: 1 in, 4 out]
                    n158 = Lossy Enqueue Element(queue=w504, element=w483) -> ()  [unwired: 1 in, 4 out]
                    n159 = And Array Elements(Boolean array=w615) -> (logical AND=w614:bool)
                    n160 = Add(x=w566, y=w567) -> (x+y=w500:dbl)
                    n161 = Lossy Enqueue Element(queue=w503, element=w477) -> ()  [unwired: 1 in, 4 out]
                    n162 = Add(x=w560, y=w561) -> (x+y=w499:dbl)
                    n163 = Lossy Enqueue Element(queue=w502, element=w475) -> ()  [unwired: 1 in, 4 out]
                    n164 = Add(x=w542, y=w543) -> (x+y=w496:dbl)
                    n165 = Add(x=w548, y=w549) -> (x+y=w497:dbl)
                    n166 = Add(x=w554, y=w555) -> (x+y=w498:dbl)
                    n167 = Add(x=w536, y=w537) -> (x+y=w495:dbl)
                    n168 = local write "系统时间"(w606) -> ()
                    n169 = Lossy Enqueue Element(queue=w494, element=w500) -> ()  [unwired: 1 in, 4 out]
                    n170 = Lossy Enqueue Element(queue=w493, element=w499) -> ()  [unwired: 1 in, 4 out]
                    n171 = Lossy Enqueue Element(queue=w491, element=w497) -> ()  [unwired: 1 in, 4 out]
                    n172 = Lossy Enqueue Element(queue=w485, element=w487) -> ()  [unwired: 1 in, 4 out]
                    n173 = Lossy Enqueue Element(queue=w492, element=w498) -> ()  [unwired: 1 in, 4 out]
                    n174 = Lossy Enqueue Element(queue=w489, element=w495) -> ()  [unwired: 1 in, 4 out]
                    n175 = Lossy Enqueue Element(queue=w490, element=w496) -> ()  [unwired: 1 in, 4 out]
                    n176 = Lossy Enqueue Element(queue=w486, element=w488) -> ()  [unwired: 1 in, 4 out]
                    n177 = case shown="真" w614 {
                      tunnel: [w638 w657] -> w612
                      tunnel: [TRUE FALSE] -> w613
                      tunnel: w602 -> [w636 w657]
                      tunnel: w482 -> [_ w656]
                      tunnel: w478 -> [_ w655]
                      tunnel: w476 -> [_ w654]
                      tunnel: w474 -> [_ w653]
                      tunnel: w505 -> [_ w652]
                      tunnel: w601 -> [w634 w650]
                      tunnel: [w634 w649] -> w600
                      tunnel: w599 -> [w635 w648]
                      tunnel: [w635 w647] -> w598
                      tunnel: w597 -> [w633 w646]
                      tunnel: [w633 w645] -> w596
                      tunnel: w529 -> [w632 w644]
                      tunnel: [w632 w643] -> w595
                      tunnel: [w631 w642] -> w594
                      tunnel: w593 -> [w631 w641]
                      tunnel: w591 -> [_ w640]
                      tunnel: [FALSE w639] -> w589
                      frame False {
                        n178 = TCP Close Connection(connection ID=w636) -> (connection ID out=w638:refnum<k5>)  [unwired: 2 in, 1 out]
                      }
                      frame True {
                        n179 = case shown="真" w640 {
                          tunnel: w656 -> [_ w710]
                          tunnel: w655 -> [_ w690]
                          tunnel: w654 -> [_ w689]
                          tunnel: w653 -> [_ w688]
                          tunnel: w652 -> [_ w687]
                          tunnel: w650 -> [w663 w676]
                          tunnel: [w663 w667] -> w649
                          tunnel: w648 -> [w662 w675]
                          tunnel: [w662 w674] -> w647
                          tunnel: w646 -> [w661 w673]
                          tunnel: [w661 w668] -> w645
                          tunnel: w644 -> [w660 w672]
                          tunnel: [w660 w671] -> w643
                          tunnel: [w659 w670] -> w642
                          tunnel: w641 -> [w659 w669]
                          tunnel: [FALSE w664] -> w639
                          frame False {
                          }
                          frame True {
                            n180 = local read "系统时间"() -> (w684:string)
                            n181 = local read "系统时间"() -> (w686:string)
                            n182 = local read "系统时间"() -> (w678:string)
                            n183 = local read "系统时间"() -> (w680:string)
                            n184 = local read "系统时间"() -> (w682:string)
                            n185 = String To Byte Array(string=w684) -> (unsigned byte array=w683:u8[])
                            n186 = String To Byte Array(string=w680) -> (unsigned byte array=w679:u8[])
                            n187 = String To Byte Array(string=w678) -> (unsigned byte array=w677:u8[])
                            n188 = String To Byte Array(string=w686) -> (unsigned byte array=w685:u8[])
                            n189 = String To Byte Array(string=w682) -> (unsigned byte array=w681:u8[])
                            n190 = Insert Into Array(array=w710, index=0 ("索引"), new element=w677) -> (w708:i16[])
                            n191 = Insert Into Array(array=w690, index=0 ("索引"), new element=w679) -> (w704:i16[])
                            n192 = Insert Into Array(array=w689, index=0 ("索引"), new element=w681) -> (w700:i16[])
                            n193 = Insert Into Array(array=w688, index=0 ("索引"), new element=w683) -> (w696:i16[])
                            n194 = Insert Into Array(array=w687, index=0 ("索引"), new element=w685) -> (w692:u16[])
                            n195 = Write to Binary File(file (use dialog)=w676, data=w708, 5:FALSE ("预置数组或字符串大小？(T)"), 9:T2."little-endian" ("字节顺序(0:big-endian, network order)")) -> (refnum out=w667:refnum<file>)  [unwired: 2 in, 2 out]
                            n196 = Write to Binary File(file (use dialog)=w675, data=w704, 5:FALSE ("预置数组或字符串大小？(T)"), 9:T2."little-endian" ("字节顺序(0:big-endian, network order)")) -> (refnum out=w674:refnum<file>)  [unwired: 2 in, 2 out]
                            n197 = Write to Binary File(file (use dialog)=w673, data=w700, 5:FALSE ("预置数组或字符串大小？(T)"), 9:T2."little-endian" ("字节顺序(0:big-endian, network order)")) -> (refnum out=w668:refnum<file>)  [unwired: 2 in, 2 out]
                            n198 = Write to Binary File(file (use dialog)=w672, data=w696, 5:FALSE ("预置数组或字符串大小？(T)"), 9:T2."little-endian" ("字节顺序(0:big-endian, network order)")) -> (refnum out=w671:refnum<file>)  [unwired: 2 in, 2 out]
                            n199 = Write to Binary File(file (use dialog)=w669, data=w692, 5:FALSE ("预置数组或字符串大小？(T)"), 9:T2."little-endian" ("字节顺序(0:big-endian, network order)")) -> (refnum out=w670:refnum<file>)  [unwired: 2 in, 2 out]
                            n200 = Get File Size(file=w667) -> (size (in bytes)=w666:i64)  [unwired: 1 in, 2 out]
                            n201 = Greater Or Equal?(x=w666, y=i64 60000000) -> (x >= y?=w664:bool)
                          }
                        }
                      }
                    }
                  }
                }
              }
            }
          }
        }
      }
    }
    n202 = Divide(x=u8 211, y=w214) -> (x/y=w212:dbl)
    n203 = Round Toward -Infinity(1:w212) -> (0:w216:dbl)
    n204 = Multiply(x=w216, y=500.0) -> (x*y=w215:dbl)
    n205 = Quotient & Remainder(x=w233, y=w216) -> (x-y*floor(x/y)=w232:dbl)  [unwired: 1 out]
    n206 = Equal?(x=w232, y=0) -> (x = y?=w230:bool)
    n207 = case shown="真" w230 {
      tunnel: w229 -> [w270 w299]
      tunnel: w228 -> [w269 w298]
      tunnel: w227 -> [w268 w297]
      tunnel: w226 -> [w267 w296]
      tunnel: [w278 w299] -> w219
      tunnel: [w277 w298] -> w220
      tunnel: [w276 w297] -> w221
      tunnel: [w275 w296] -> w222
      tunnel: w218 -> [w274 w292]
      tunnel: w225 -> [w273 w295]
      tunnel: w224 -> [w272 w293]
      tunnel: w223 -> [w271 w294]
      tunnel: w215 -> [_ w291]
      tunnel: w206 -> [_ w286]
      tunnel: w205 -> [_ w285]
      tunnel: w204 -> [_ w284]
      tunnel: w203 -> [_ w283]
      frame False {
        n208 = Array Size(array=w273) -> (size(s)=w280:i32)
        n209 = Array Size(array=w274) -> (size(s)=w279:i32)
        n210 = Array Size(array=w271) -> (size(s)=w282:i32)
        n211 = Array Size(array=w272) -> (size(s)=w281:i32)
        n212 = Insert Into Array(array=w273, index=w280, new element=w268) -> (w276:dbl[])
        n213 = Insert Into Array(array=w274, index=w279, new element=w267) -> (w275:dbl[])
        n214 = Insert Into Array(array=w271, index=w282, new element=w270) -> (w278:dbl[])
        n215 = Insert Into Array(array=w272, index=w281, new element=w269) -> (w277:dbl[])
      }
      frame True {
        n216 = call <vilib>:"Amplitude and Phase Spectrum.vi"("dt"=w291, "Signal (V)"=w293) -> ("Amp Spectrum Mag (Vrms)"=w288:dbl[])  [unwired: 1 in, 2 out]
        n217 = call <vilib>:"Amplitude and Phase Spectrum.vi"("dt"=w291, "Signal (V)"=w292) -> ("Amp Spectrum Mag (Vrms)"=w290:dbl[])  [unwired: 1 in, 2 out]
        n218 = call <vilib>:"Amplitude and Phase Spectrum.vi"("dt"=w291, "Signal (V)"=w294) -> ("Amp Spectrum Mag (Vrms)"=w287:dbl[])  [unwired: 1 in, 2 out]
        n219 = call <vilib>:"Amplitude and Phase Spectrum.vi"("dt"=w291, "Signal (V)"=w295) -> ("Amp Spectrum Mag (Vrms)"=w289:dbl[])  [unwired: 1 in, 2 out]
        n220 = Lossy Enqueue Element(queue=w286, element=w290) -> ()  [unwired: 1 in, 4 out]
        n221 = Lossy Enqueue Element(queue=w284, element=w288) -> ()  [unwired: 1 in, 4 out]
        n222 = Lossy Enqueue Element(queue=w283, element=w287) -> ()  [unwired: 1 in, 4 out]
        n223 = Lossy Enqueue Element(queue=w285, element=w289) -> ()  [unwired: 1 in, 4 out]
      }
    }
    n224 = Dequeue Element(queue=w188) -> (element=w189:bool)  [unwired: 2 in, 3 out]
    n225 = Add(x=w265, y=w247) -> (x+y=w266:i32)
    "收包" <- w266
    n226 = Tick Count (ms)() -> (millisecond timer value=w257:u32)
    n227 = Subtract(x=w257, y=w258) -> (x-y=w256:u32)
    n228 = Not(x=w189) -> (.not. x?=w190:bool)
    n229 = Subtract(x=w266, y=w265) -> (x-y=w264:i32)
    n230 = Add(x=w264, y=w263) -> (x+y=w259:i32)
    n231 = Add(x=w253, y=w256) -> (x+y=w254:u32)
    n232 = Greater Or Equal?(x=w259, y=1000000) -> (x >= y?=w261:bool)
    n233 = Compound Arithmetic op=OR(w192, w191, w190) -> (w193:bool)
    n234 = case shown="真" w261 {
      tunnel: [w713 0] -> w260
      tunnel: w259 -> [w713 w716]
      tunnel: [w712 u32 0] -> w255
      tunnel: w254 -> [w712 w717]
      frame False {
      }
      frame True {
        n235 = Divide(x=w716, y=w717) -> (x/y=→"KB/s":dbl)
      }
    }
  }
  n236 = TCP Close Connection(connection ID=w2) -> ()  [unwired: 2 in, 2 out]
